vi "Parse Config.vi"(8 "error in (no error)":errorcluster, 10 "Config String":string, 11 "SPI Root Pattern Creator in":refnum<class "SPI Root Pattern Creator.lvclass">) -> (0 "error out":errorcluster, 3 "SPI Root Pattern Creator out":refnum<class "SPI Root Pattern Creator.lvclass">)   [LabVIEW 2018, in "SPI Root Pattern Creator.lvlib" / "SPI Root Pattern Creator.lvclass"]
uses:
  SPI Root Pattern Creator.lvclass
  Ctls/Frame Data - SPI_3W.ctl
  Ctls/RW Options.ctl
  SPI Root Pattern Creator.lvclass/SPI Root Pattern Creator.ctl
  Write FRM Data.vi
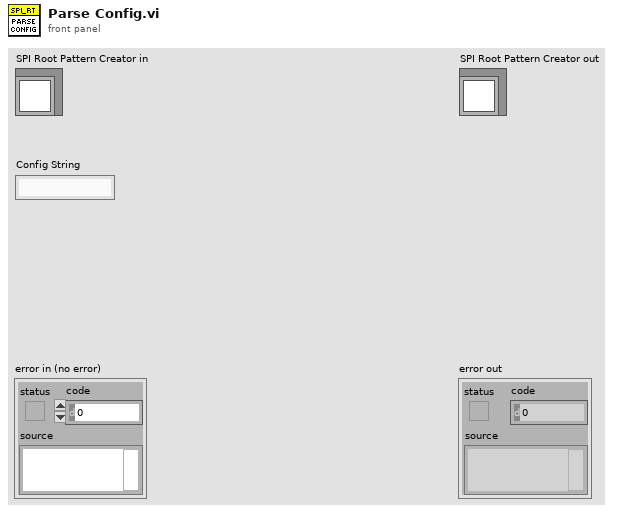
[diagram p1: front panel]
types:
  T1 = typedef "Frame Data - SPI_3W.ctl" = cluster{"Pattern Name":string, "Data":u16, "Addr":u16, "OpCode":string[], "R/W?":T2}
  T2 = typedef "RW Options.ctl" = enum16{"Read", "Write", "R/W"}
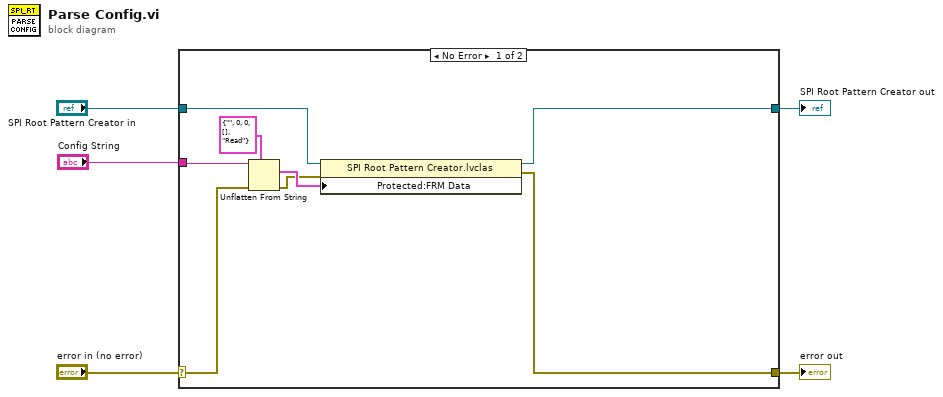
[diagram p0: block diagram]
diagram:
  n1 = case shown="No Error" "error in (no error)" {
    selector: "error in (no error)" -> [w12 w15]
    tunnel: [w6 w15] -> w4
    tunnel: [w7 w14] -> w2
    tunnel: "SPI Root Pattern Creator in" -> [w10 w14]
    tunnel: "Config String" -> [w13 _]
    frame No Error {
      n2 = Unflatten From String(type=T1 {"Pattern Name"="", "Data"=0, "Addr"=0, "OpCode"=[], "R/W?"=enum."Read"} ("FRM Data"), binary string=w13, error in (no error)=w12) -> (value=w9:T1, error out=w8:errorcluster)  [unwired: 2 in, 1 out]
      n3 = property class="SPI Root Pattern Creator.lvclas"(reference=w10, error in=w8, "Protected:FRM Data"=w9) -> (reference out=w7:refnum<class "SPI Root Pattern Creator.lvclass">, error out=w6:errorcluster)
    }
    frame Error {
    }
  }
  "error out" <- w4
  "SPI Root Pattern Creator out" <- w2
